vi "Stop Acquisition and Logging.vi"(8 "error in (no error)":errorcluster, 11 "FPGA VI Reference":T1) -> (0 "error out":errorcluster, 3 "Stop FPGA Timeout?":bool)   [LabVIEW 2020]
doc: "This VI sends a stop command to the FPGA's acquisition loop and waits for confirmation that the loop has indeed stopped. The VI also flushes the UI's data buffer so subsequent acquisitions do not read old data."
uses:
  controls/FPGA VI Reference.ctl
  <vilib>/Utility/error.llb/Error Cluster From Error Code.vi
  <vilib>/rvi/errors/niLvFpgaAdjustHostInterfaceError.vi
  <vilib>/FPGAPlugInAG/cRIO-9038/niLvFpga_Close_cRIO-9038.vi
  <vilib>/rvi/interface/nirviReadWriteControl/nirviReadWriteControl.xnode
  FPGA Bitfiles/forthexerciseemc_FPGATarget2_FPGAMain_d5JOh9LSVOQ.lvbitx
  <vilib>/rvi/interface/nirviMethod/nirviMethod.xnode
  <vilib>/rvi/interface/nirviCloseFPGA/nirviCloseFPGA.xnode
  <vilib>/rvi/errors/niLvFpgaMergeErrorWithErrorCode.vi
  NiFpgaLv.dll
  <vilib>/FPGAPlugInAG/cRIO-9038/niLvFpga_ReadFifo_cRIO-9038.vi
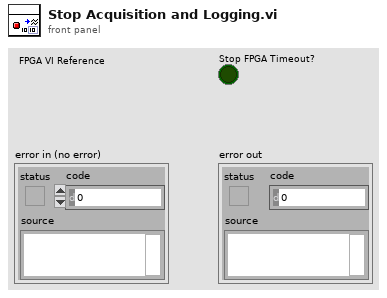
[diagram p1: front panel]
types:
  T1 = typedef "FPGA VI Reference.ctl" = refnum<k20>
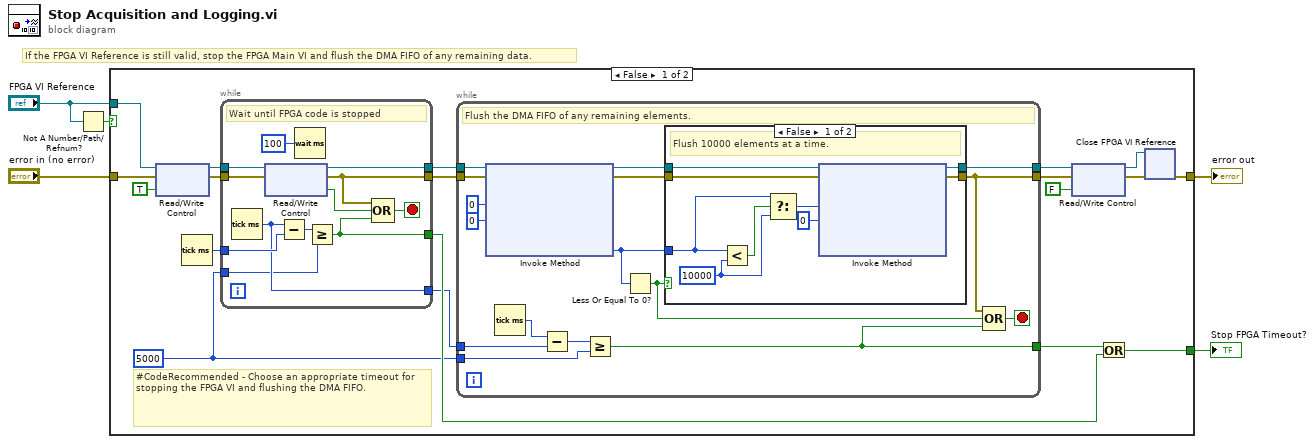
[diagram p0: block diagram]
diagram:
  # "If the FPGA VI Reference is still valid, stop the FPGA Main VI and flush the DMA FIFO of any remaining data."
  n1 = Not A Number/Path/Refnum?(number/path/refnum="FPGA VI Reference") -> (NaN/Path/Refnum?=w2:bool)
  n2 = case shown="False" w2 {
    tunnel: [w10 w64] -> w5
    tunnel: "FPGA VI Reference" -> [w9 _]
    tunnel: "error in (no error)" -> [w8 w64]
    tunnel: [w6 _] -> w1
    frame False {
      w7 = u32 5000 ("y")
      # "#CodeRecommended - Choose an appropriate timeout for stopping the FPGA VI and flushing the DMA FIFO."
      n3 = xnode "Read/Write Control"("FPGA VI Reference In"=w9, "error in"=w8, "Stop"=TRUE) -> ("FPGA VI Reference Out"=w22:T1, "error out"=w21:errorcluster)
      n4 = Tick Count (ms)() -> (millisecond timer value=w16:u32)
      n5 = while {
        tunnel: w22 -> [w63]
        tunnel: w21 -> [w62]
        tunnel: [w60] -> w20
        tunnel: [w52] -> w19
        tunnel: w16 -> [w59]
        tunnel: [w55] -> w14
        tunnel: [w54] -> w13
        tunnel: w7 -> [w53]
        stop <- w57 stop-if-true
        # "Wait until FPGA code is stopped"
        n6 = Tick Count (ms)() -> (millisecond timer value=w54:u32)
        n7 = xnode "Read/Write Control"("FPGA VI Reference In"=w63, "error in"=w62) -> ("FPGA VI Reference Out"=w60:T1, "error out"=w52:errorcluster, "Finished"=w56:bool)
        n8 = Subtract(x=w54, y=w59) -> (x-y=w58:u32)
        n9 = Wait (ms)(milliseconds to wait=u32 100) -> ()  [unwired: 1 out]
        n10 = Greater Or Equal?(x=w58, y=w53) -> (x >= y?=w55:bool)
        n11 = Compound Arithmetic op=OR(w52, w56, w55) -> (w57:bool)
      }
      n12 = while {
        tunnel: [w37] -> w18
        tunnel: [w25] -> w17
        tunnel: w20 -> [w35]
        tunnel: w19 -> [w34]
        tunnel: w13 -> [w28]
        tunnel: [w27] -> w15
        tunnel: w7 -> [w26]
        stop <- w32 stop-if-true
        # "Flush the DMA FIFO of any remaining elements."
        n13 = xnode "Invoke Method"("FPGA VI Reference In"=w35, "error in"=w34, "Number of Elements"=u32 0, "Timeout (ms)"=0) -> ("FPGA VI Reference Out"=w40:T1, "error out"=w39:errorcluster, "Elements Remaining"=w33:u32)  [unwired: 1 out]
        n14 = Tick Count (ms)() -> (millisecond timer value=w29:u32)
        n15 = Subtract(x=w29, y=w28) -> (x-y=w30:u32)
        n16 = Greater Or Equal?(x=w30, y=w26) -> (x >= y?=w27:bool)
        n17 = Less Or Equal To 0?(x=w33) -> (x <= 0?=w31:bool)
        n18 = case shown="False" w31 {
          tunnel: w40 -> [w49 w51]
          tunnel: w39 -> [w48 w50]
          tunnel: [w46 w51] -> w37
          tunnel: [w45 w50] -> w25
          tunnel: w33 -> [w41 _]
          frame False {
            w43 = u32 10000
            # "Flush 10000 elements at a time."
            n19 = Less?(x=w41, y=w43) -> (x < y?=w44:bool)
            n20 = Select(t=w41, s=w44, f=w43) -> (s? t:f=w42:u32)
            n21 = xnode "Invoke Method"("FPGA VI Reference In"=w49, "error in"=w48, "Number of Elements"=w42, "Timeout (ms)"=0) -> ("FPGA VI Reference Out"=w46:T1, "error out"=w45:errorcluster)  [unwired: 2 out]
          }
          frame True {
            # "Buffer is empty"
          }
        }
        n22 = Compound Arithmetic op=OR(w25, w31, w27) -> (w32:bool)
      }
      n23 = xnode "Read/Write Control"("FPGA VI Reference In"=w18, "error in"=w17, "Stop"=FALSE) -> ("FPGA VI Reference Out"=w12:T1, "error out"=w11:errorcluster)
      n24 = Or(x=w15, y=w14) -> (x .or. y?=w6:bool)
      n25 = xnode "Close FPGA VI Reference"("FPGA VI Reference In"=w12, "error in"=w11) -> ("error out"=w10:errorcluster)
    }
    frame True {
    }
  }
  "error out" <- w5
  "Stop FPGA Timeout?" <- w1
